vi "Delete Number of Lines.vi"(7 "Position":enum16{"Top", "Bottom", "Line N"}(ring), 9 "Line Terminator (\\n)":string="\n", 10 "Number of Lines":i32, 11 "String":string) -> (3 "Resulting String":string)   [LabVIEW 2020]
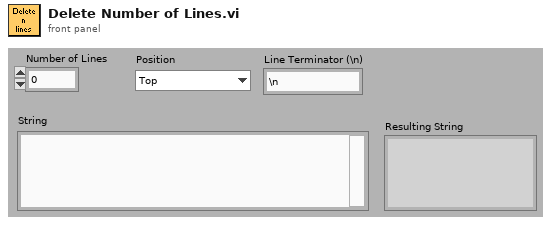
[diagram p1: front panel]
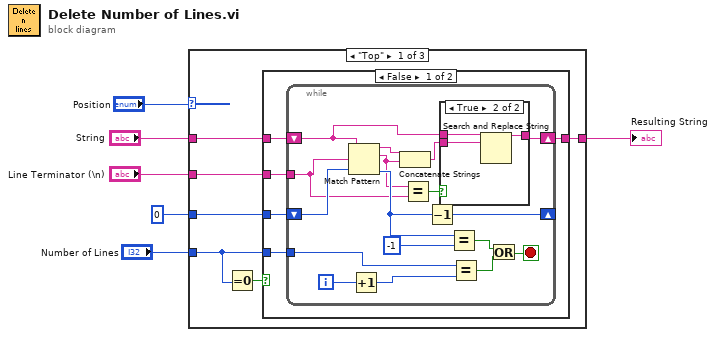
[diagram p0: block diagram]
diagram:
  n1 = case shown="\"Top\"" "Position" {
    tunnel: "String" -> [w10 w40 w41]
    tunnel: 0 ("offset past token") -> [w12 _ _]
    tunnel: "Line Terminator (\\n)" -> [w11 _ _]
    tunnel: [w9 w40 w41] -> w2
    tunnel: "Number of Lines" -> [w7 _ _]
    frame "Top" {
      n2 = Equal To 0?(x=w7) -> (x = 0?=w8:bool)
      n3 = case shown="False" w8 {
        tunnel: w12 -> [w17 _]
        tunnel: w11 -> [w16 _]
        tunnel: w10 -> [w15 w39]
        tunnel: [w14 w39] -> w9
        tunnel: w7 -> [w13 _]
        frame False {
          n4 = while {
            shift-right: [w18] -> _
            shift-left: w17 -> [w34]
            tunnel: w16 -> [w28]
            shift-right: [w31] -> w14
            shift-left: w15 -> [w30]
            tunnel: w13 -> [w24]
            i -> [w25]
            stop <- w27 stop-if-true
            n5 = Match Pattern(string=w30, regular expression=w28, offset (0)=w34) -> (before substring=w20:string, match substring=w21:string, offset past match=w32:i32)  [unwired: 1 out]
            n6 = Increment(x=w25) -> (x+1=w23:i32)
            n7 = Concatenate Strings(w20, w21) -> (w19:string)
            n8 = Equal?(x=w21, y=w28) -> (x = y?=w29:bool)
            n9 = Decrement(x=w32) -> (x-1=w18:i32)
            n10 = case shown="True" w29 {
              tunnel: w19 -> [_ w38]
              tunnel: [w35 w37] -> w31
              tunnel: w30 -> [w35 w36]
              frame False {
              }
              frame True {
                n11 = Search and Replace String(input string=w36, search string=w38) -> (result string=w37:string)  [unwired: 6 in, 3 out]
              }
            }
            n12 = Equal?(x=w32, y=-1) -> (x = y?=w26:bool)
            n13 = Equal?(x=w24, y=w23) -> (x = y?=w22:bool)
            n14 = Or(x=w26, y=w22) -> (x .or. y?=w27:bool)
          }
        }
        frame True {
        }
      }
    }
    frame "Bottom" {
    }
    frame "Line N" {
    }
  }
  "Resulting String" <- w2
